vi "Read_Instr.vi"(8 "error in (no error)":errorcluster caption="entrée d'erreur (pas d'erreur)", 11 "Class Instrument (Default) en entrée":refnum<class "Class Instrument Printer.lvclass">) -> (0 "error out":errorcluster caption="sortie d'erreur", 3 "Class Instrument (Default) en sortie":refnum<class "Class Instrument Printer.lvclass">)   [LabVIEW 2020, in "Library Instrument & Equipement.lvlib" / "Library Instruments.lvlib" / "Class Instrument Printer.lvclass"]
uses:
  Class Instrument Printer.lvclass
  Commun VI/TypeDef/Liste Error.ctl
  Instrument (Default)/Class Instrument (Default).lvclass
  Commun VI/Library Commun.lvlib
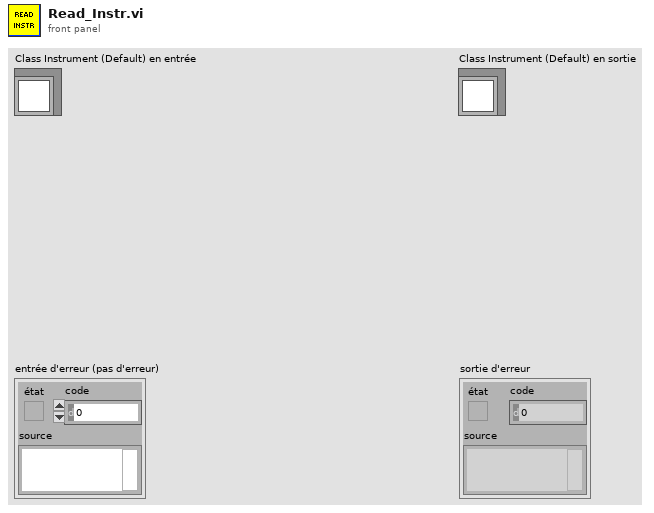
[diagram p1: front panel]
types:
  T1 = typedef "Library Commun.lvlib/Liste Error.ctl" = enum16{"Firebase Driver - Get Document", "Firebase Driver - Get Document With Where", "Firebase Driver - Delete Document", "Firebase Driver - Set Document", "Firebase Driver - Update Document", "Firebase Altyor - Search Document Bench", "Firebase Altyor - Class Not in Firebase", "Spectrum_Analyser - Timeout", "Relay Board - Qty Relay", "DIO - Pb Funtion", "Power_Supply - Peripherical not find", "Mutimeter - Peripherical not find", "Instrument - Function Not Used", "Instrument - Instrument name not specified", "Instrument - Allready Initialised", "Instrument - TimeOut", "Instrument - the instrument must be Initialise before", "Instrument - Frame Not received", "Instrument - Frame Nok", "Test - Initialise the File_for_Save", "Test - Timeout", "Test - Cmd Error", "FGV - Variable ", "BDD FireBase - Define Class", "SN - Class Not Define"}
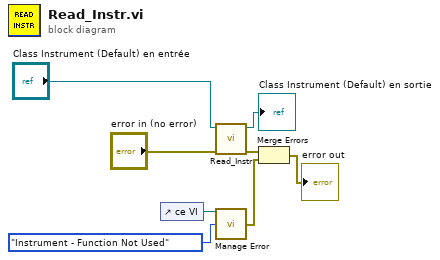
[diagram p0: block diagram]
diagram:
  n1 = control-ref of="ce VI"() -> (w8:refnum<vi>)
  n2 = call-parent "Read_Instr.vi"("error in (no error)"="error in (no error)", "Class Instrument (Default) en entrée"="Class Instrument (Default) en entrée") -> ("error out"=w5:errorcluster, "Class Instrument (Default) en sortie"=→"Class Instrument (Default) en sortie":refnum<class "Class Instrument Printer.lvclass">)  [unwired: 8 in]
  n3 = call "Manage Error.vi"("VI in Error"=w8, "Code Erreur"=Liste_Error."Instrument - Function Not Used") -> ("error out"=w4:errorcluster)  [unwired: 13 in]
  n4 = Merge Errors(w5, w4) -> (→"error out":errorcluster)
